vi "Write R shunt.vi"(8 "error in (no error)":errorcluster, 10 "R shunt":dbl, 11 "Heat Flow Results in":refnum<class "Heat Flow Results.lvclass">) -> (0 "error out":errorcluster, 3 "Heat Flow Results out":refnum<class "Heat Flow Results.lvclass">)   [LabVIEW 2019, in "Results.lvlib" / "Heat Flow Results.lvclass"]
uses:
  Heat Flow Results.lvclass
  Heat Flow Results.lvclass/Heat Flow Results.ctl
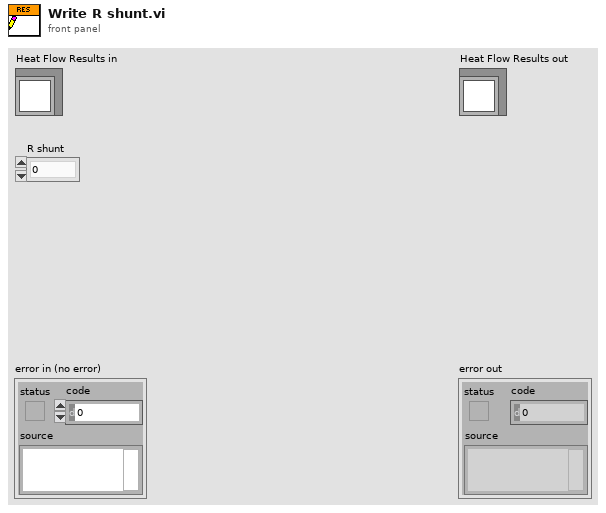
[diagram p1: front panel]
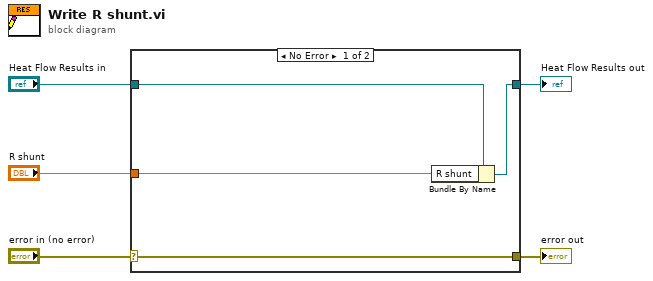
[diagram p0: block diagram]
diagram:
  n1 = case shown="No Error" "error in (no error)" {
    selector: "error in (no error)" -> [w9 w10]
    tunnel: [w9 w10] -> w4
    tunnel: [w7 w11] -> w2
    tunnel: "Heat Flow Results in" -> [w8 w11]
    tunnel: "R shunt" -> [w6 _]
    frame No Error {
      n2 = Bundle By Name(cluster=w8, "R shunt"=w6) -> (w7:refnum<class "Heat Flow Results.lvclass">)
    }
    frame Error {
    }
  }
  "error out" <- w4
  "Heat Flow Results out" <- w2
